vi "Width Fixer on modules Selector.vi"(9 "Left":i16, 10 "Right":i16, 11 "VI in":refnum<vi>) -> ()   [LabVIEW 2019, in "Panther Dashboard.lvlib"]
uses:
  Panther Dashboard.lvlib
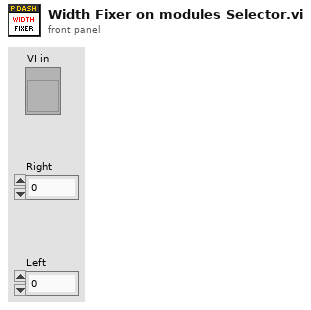
[diagram p1: front panel]
types:
  T1 = typedef "LVRectTypeDef.ctl" = cluster{"Left":i16, "Top":i16, "Right":i16, "Bottom":i16}
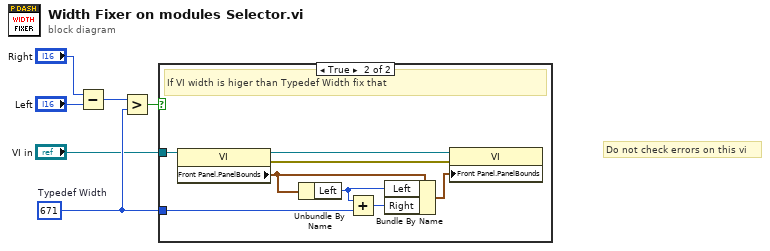
[diagram p0: block diagram]
diagram:
  w6 = i16 671  # Typedef Width
  # "Do not check errors on this vi"
  n1 = Subtract(x="Right", y="Left") -> (x-y=w3:i16)
  n2 = Greater?(x=w3, y=w6) -> (0:w4:bool)
  n3 = case shown="True" w4 {
    tunnel: "VI in" -> [_ w13]
    tunnel: w6 -> [_ w8]
    frame False {
    }
    frame True {
      # "If VI width is higer than Typedef Width fix that"
      n4 = property class="VI"(reference=w13) -> (reference out=w12:refnum<vi>, error out=w14:errorcluster, "Front Panel.PanelBounds"=w11:T1)  [unwired: 1 in]
      n5 = Unbundle By Name(w11) -> ("Left"=w9:i16)
      n6 = Add(x=w9, y=w8) -> (x+y=w7:i16)
      n7 = Bundle By Name(cluster=w11, "Left"=w9, "Right"=w7) -> (w10:T1)
      n8 = property class="VI"(reference=w12, error in=w14, "Front Panel.PanelBounds"=w10) -> ()  [unwired: 2 out]
    }
  }
